vi "drive to boiler.vi"() -> (1 "y output":dbl, 3 "x output":dbl)   [LabVIEW 2016]
uses:
  Robot Global Data.vi
panel:
  out "%error":dbl
  out "sees boiler":bool
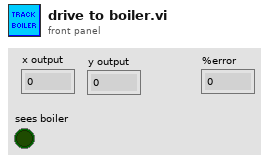
[diagram p1: front panel]
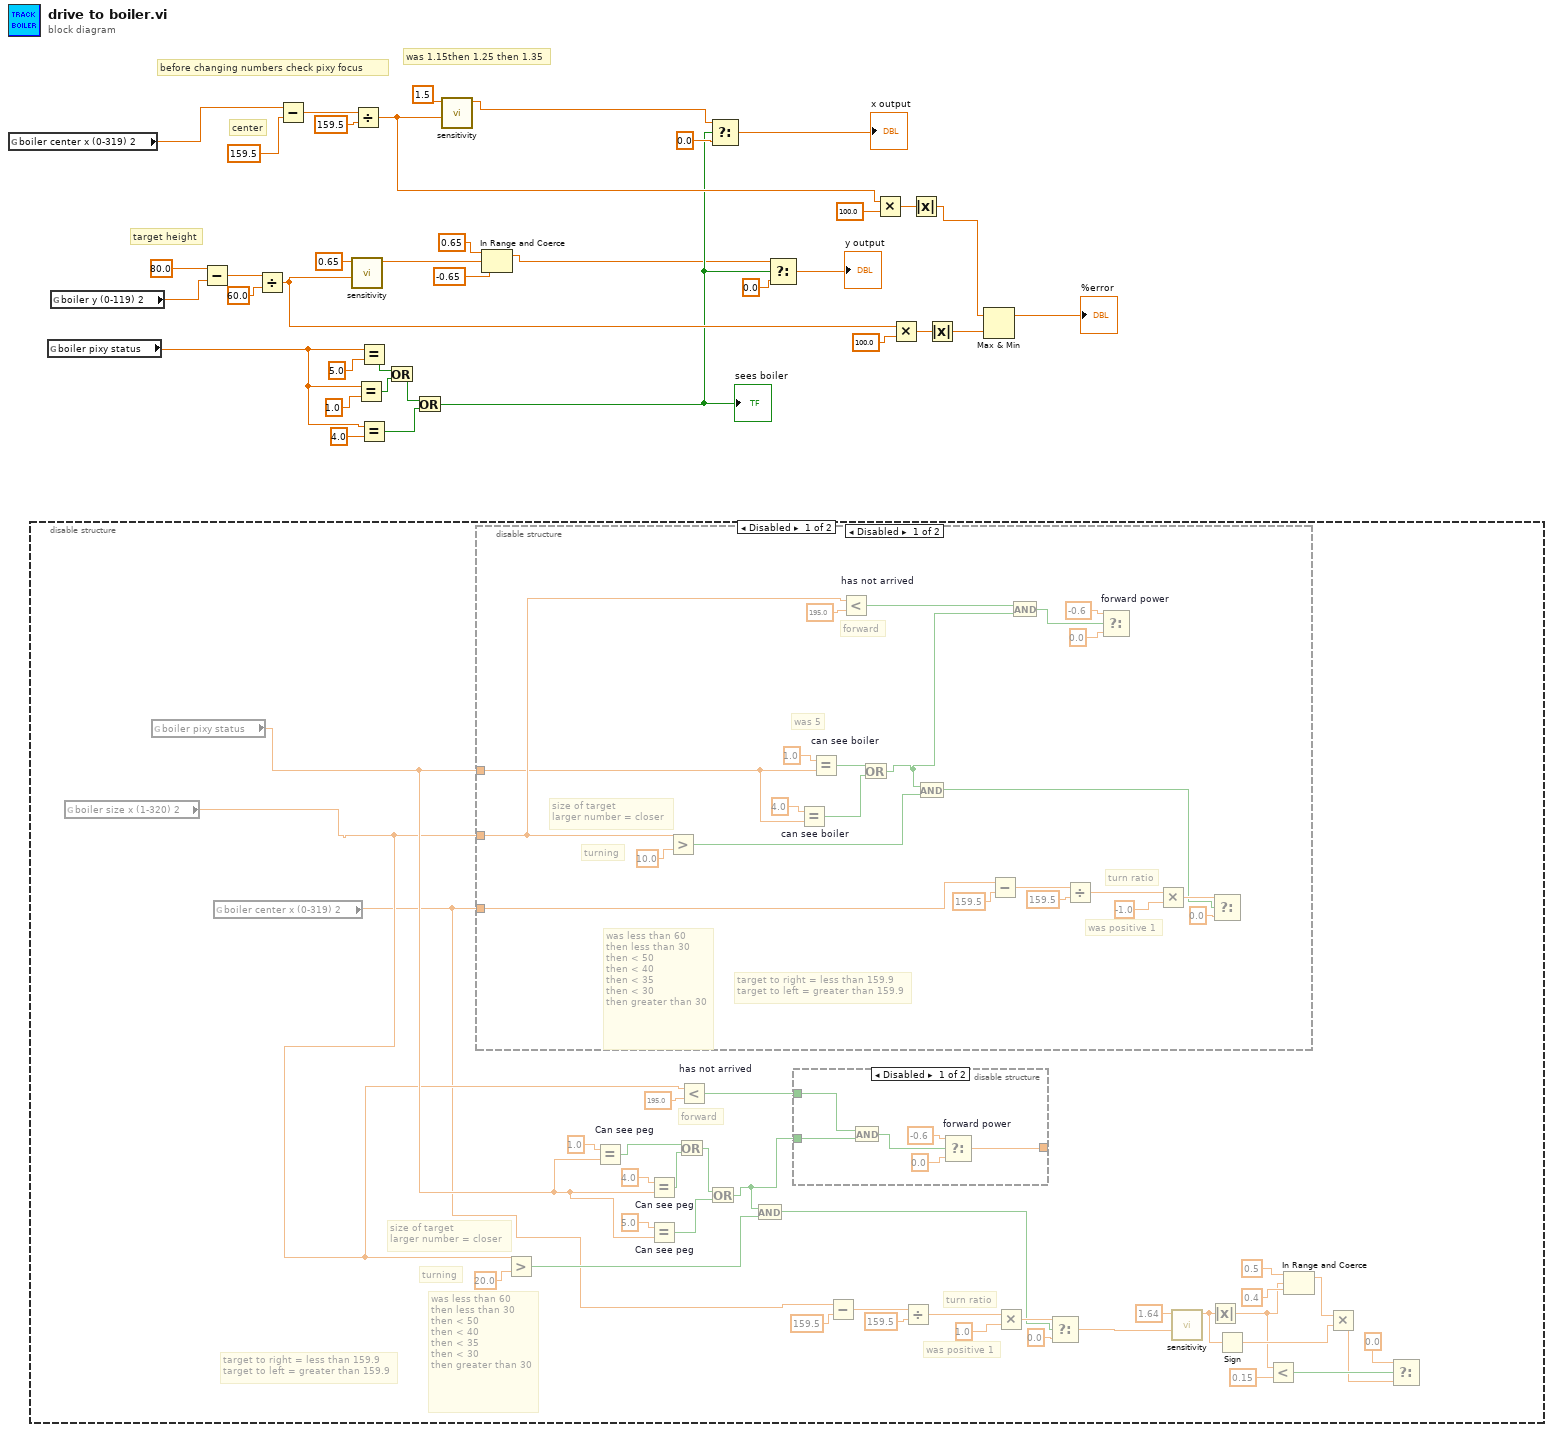
[diagram p0: block diagram]
diagram:
  # "was 1.15then 1.25 then 1.35"
  # "center"
  # "target height"
  # "before changing numbers check pixy focus"
  n1 = global read "Robot Global Data.vi" "boiler center x (0-319) 2"() -> (w33:dbl)
  n2 = disable-structure shown="Disabled" {
    frame Disabled {
      # "forward"
      # "was positive 1"
      # "turning"
      # "size of target\nlarger number = closer"
      # "turn ratio"
      # "was less than 60\nthen less than 30\nthen < 50\nthen < 40\nthen < 35\nthen < 30\nthen greater than 30"
      # "target to right = less than 159.9\ntarget to left = greater than 159.9"
      n3 = global read "Robot Global Data.vi" "boiler size x (1-320) 2"() -> (w39:dbl)
      n4 = global read "Robot Global Data.vi" "boiler pixy status"() -> (w40:dbl)
      n5 = global read "Robot Global Data.vi" "boiler center x (0-319) 2"() -> (w38:dbl)
      n6 = disable-structure shown="Disabled" {
        disable-tunnel: w38 -> [w94 _]
        disable-tunnel: w39 -> [w93 _]
        disable-tunnel: w40 -> [w91 _]
        frame Disabled {
          # "target to right = less than 159.9\ntarget to left = greater than 159.9"
          # "forward"
          # "was 5"
          # "was positive 1"
          # "turning"
          # "size of target\nlarger number = closer"
          # "turn ratio"
          # "was less than 60\nthen less than 30\nthen < 50\nthen < 40\nthen < 35\nthen < 30\nthen greater than 30"
          n7 = Greater?(x=w93, y=10.0) -> (0:w97:bool)
          n8 = Equal? "can see boiler"(x=4.0 ("y"), y=w91) -> (x = y?=w89:bool)
          n9 = Equal? "can see boiler"(x=1.0 ("y"), y=w91) -> (x = y?=w90:bool)
          n10 = Less? "has not arrived"(x=w93, y=195.0) -> (x < y?=w82:bool)
          n11 = Or(x=w90, y=w89) -> (x .or. y?=w88:bool)
          n12 = And(x=w88, y=w97) -> (x .and. y?=w98:bool)
          n13 = Subtract(x=w94, y=159.5) -> (x-y=w104:dbl)
          n14 = And(x=w82, y=w88) -> (x .and. y?=w84:bool)
          n15 = Divide(x=w104, y=159.5) -> (x/y=w100:dbl)
          n16 = Select "forward power"(t=-0.6, s=w84, f=0.0) -> (s? t:f=w81:dbl)
          n17 = Multiply(x=w100, y=-1.0) -> (x*y=w101:dbl)
          n18 = Select(t=w101, s=w98, f=0.0) -> (s? t:f=w95:dbl)
        }
        frame Enabled {
        }
      }
      n19 = Greater?(x=w39, y=20.0) -> (0:w64:bool)
      n20 = Equal? "Can see peg"(x=1.0 ("y"), y=w40) -> (x = y?=w58:bool)
      n21 = Equal? "Can see peg"(x=4.0 ("y"), y=w40) -> (x = y?=w56:bool)
      n22 = Equal? "Can see peg"(x=5.0 ("y"), y=w40) -> (x = y?=w55:bool)
      n23 = Or(x=w58, y=w56) -> (x .or. y?=w54:bool)
      n24 = Less? "has not arrived"(x=w39, y=195.0) -> (x < y?=w63:bool)
      n25 = Or(x=w54, y=w55) -> (x .or. y?=w53:bool)
      n26 = And(x=w53, y=w64) -> (x .and. y?=w66:bool)
      n27 = disable-structure shown="Disabled" {
        disable-tunnel: w63 -> [w77 _]
        disable-tunnel: [w76 _] -> w61
        disable-tunnel: w53 -> [w75 _]
        frame Disabled {
          n28 = And(x=w77, y=w75) -> (x .and. y?=w78:bool)
          n29 = Select "forward power"(t=-0.6, s=w78, f=0.0) -> (s? t:f=w76:dbl)
        }
        frame Enabled {
        }
      }
      n30 = Subtract(x=w38, y=159.5) -> (x-y=w72:dbl)
      n31 = Divide(x=w72, y=159.5) -> (x/y=w68:dbl)
      n32 = Multiply(x=w68, y=1.0) -> (x*y=w69:dbl)
      n33 = Select(t=w69, s=w66, f=0.0) -> (s? t:f=w60:dbl)
      n34 = call "sensitivity.vi"("x"=w60, "sensitivity"=1.64) -> ("scaled value"=w49:dbl)  [unwired: 9 in]
      n35 = Absolute Value(x=w49) -> (abs(x)=w46:dbl)
      n36 = Sign(1:w49) -> (0:w47:dbl)
      n37 = Less?(x=w46, y=0.15) -> (x < y?=w44:bool)
      n38 = In Range and Coerce(upper limit=0.5, x=w46, lower limit=0.4) -> (coerced(x)=w48:dbl)  [unwired: 1 out]
      n39 = Multiply(x=w48, y=w47) -> (x*y=w43:dbl)
      n40 = Select(t=0.0, s=w44, f=w43) -> (s? t:f=w41:dbl)
    }
    frame Enabled {
    }
  }
  n41 = global read "Robot Global Data.vi" "boiler pixy status"() -> (w25:dbl)
  n42 = global read "Robot Global Data.vi" "boiler y (0-119) 2"() -> (w5:dbl)
  n43 = Subtract(x=80.0 ("y"), y=w5) -> (x-y=w21:dbl)
  n44 = Divide(x=w21, y=60.0) -> (x/y=w18:dbl)
  n45 = Subtract(x=w33, y=159.5) -> (x-y=w36:dbl)
  n46 = call "sensitivity.vi"("x"=w18, "sensitivity"=0.65) -> ("scaled value"=w4:dbl)  [unwired: 9 in]
  n47 = Divide(x=w36, y=159.5) -> (x/y=w10:dbl)
  n48 = Equal?(x=w25, y=1.0) -> (x = y?=w28:bool)
  n49 = Equal?(x=w25, y=5.0) -> (x = y?=w29:bool)
  n50 = Equal?(x=w25, y=4.0) -> (x = y?=w23:bool)
  n51 = Or(x=w29, y=w28) -> (x .or. y?=w22:bool)
  n52 = Or(x=w22, y=w23) -> (x .or. y?=w7:bool)
  "sees boiler" <- w7
  n53 = call "sensitivity.vi"("x"=w10, "sensitivity"=1.5) -> ("scaled value"=w27:dbl)  [unwired: 9 in]
  n54 = In Range and Coerce(upper limit=0.65, x=w4, lower limit=-0.65) -> (coerced(x)=w3:dbl)  [unwired: 1 out]
  n55 = Select(t=w27, s=w7, f=0.0) -> (s? t:f=→"x output":dbl)
  n56 = Select(t=w3, s=w7, f=0.0) -> (s? t:f=→"y output":dbl)
  n57 = Multiply(x=w10, y=100.0) -> (x*y=w12:dbl)
  n58 = Multiply(x=w18, y=100.0) -> (x*y=w16:dbl)
  n59 = Absolute Value(x=w12) -> (abs(x)=w11:dbl)
  n60 = Absolute Value(x=w16) -> (abs(x)=w15:dbl)
  n61 = Max & Min(x=w11, y=w15) -> (max(x,y)=→"%error":dbl)  [unwired: 1 out]
